vi "Shutdown Logging.vi"(8 "error in (no error)":errorcluster, 11 "Logging Thread in":refnum<class "Logging Thread.lvclass">) -> (0 "error out":errorcluster, 3 "Logging Thread out":refnum<class "Logging Thread.lvclass">)   [LabVIEW 2019, in "DSF Core.lvlib" / "Logging Thread.lvclass"]
uses:
  Logging Thread.lvclass
  Logging Thread.lvclass/Logging Thread.ctl
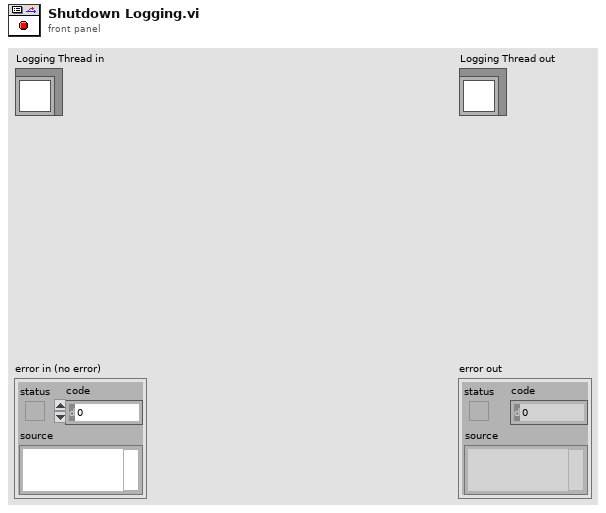
[diagram p1: front panel]
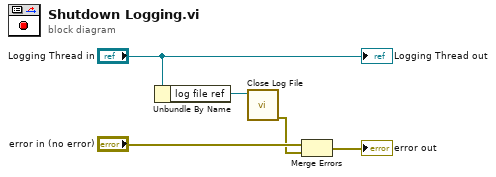
[diagram p0: block diagram]
diagram:
  n1 = Unbundle By Name("Logging Thread in") -> ("log file ref"=w5:refnum<file>)
  n2 = call "Close Log File.vi"("file refnum"=w5) -> ("error out"=w1:errorcluster)  [unwired: 10 in]
  n3 = Merge Errors("error in (no error)", w1) -> (→"error out":errorcluster)
  "Logging Thread out" <- "Logging Thread in"
